vi "Automatic.vi"() -> ()   [LabVIEW 2015]
uses:
  <vilib>/myRIO/Instrument Drivers/Onboard IO/PWM/typedefs/PWM Reference.ctl
  <vilib>/myRIO/Common/Instrument Driver Framework/Utilities/typedefs/myRIO Generic Hardware Reference.ctl
  <vilib>/myRIO/Common/Instrument Driver Framework/Utilities/typedefs/Hardware Version Enum.ctl
  <vilib>/myRIO/Common/Instrument Driver Framework/Utilities/typedefs/myRIO v1.0 Reference.ctl
  <vilib>/myRIO/Common/Instrument Driver Framework/Utilities/typedefs/Generic FPGA Reference.ctl
  <vilib>/myRIO/Common/Instrument Driver Framework/myRIO v1.0/PWM/typedefs/PWM Channels Enum.ctl
  <vilib>/myRIO/Instrument Drivers/Onboard IO/PWM/typedefs/PWM Configuration.ctl
  <vilib>/userdefined/High Color/nirio_resource_hc.ctl
  <vilib>/myRIO/Instrument Drivers/Onboard IO/DIO/typedefs/DIO Reference.ctl
  <vilib>/myRIO/Common/Instrument Driver Framework/myRIO v1.0/DIO/typedefs/DIO Channels List.ctl
  <vilib>/myRIO/Common/Instrument Driver Framework/myRIO v1.0/DIO/typedefs/DIO Channels Enum.ctl
  <vilib>/myRIO/Common/Instrument Driver Framework/Utilities/vis/Is FPGA Ref Available.vi
  <vilib>/myRIO/Common/Instrument Driver Framework/myRIO v1.0/DIO/vis/myRIO v1.1 Open DIO.vi
  <vilib>/myRIO/Instrument Drivers/Onboard IO/DIO/vis/Write.vi
  <vilib>/myRIO/Common/Instrument Driver Framework/myRIO v1.0/PWM/vis/myRIO v1.1 Open PWM.vi
  <vilib>/myRIO/Common/Instrument Driver Framework/Utilities/vis/Validate Channels.vi
  <vilib>/myRIO/Common/Instrument Driver Framework/myRIO v1.0/DIO/vis/myRIO v1.0 Reserve DIO.vi
  <vilib>/myRIO/Common/Instrument Driver Framework/myRIO v1.0/PWM/vis/myRIO v1.0 Reserve PWM.vi
  <vilib>/myRIO/Instrument Drivers/Onboard IO/PWM/vis/Set Duty Cycle and Frequency.vi
  <vilib>/myRIO/Common/Instrument Driver Framework/myRIO v1.0/PWM/vis/myRIO v1.0 Close PWM.vi
  <vilib>/myRIO/Common/Instrument Driver Framework/myRIO v1.0/UART/vis/myRIO v1.0 Close UART.vi
  <vilib>/myRIO/Common/Instrument Driver Framework/myRIO v1.0/Resource Manager/vis/myRIO v1.0 Reserve Channel List.vi
  <vilib>/myRIO/Common/Instrument Driver Framework/myRIO v1.0/DIO/vis/myRIO v1.0 Build MUX Configuration DIO.vi
  <vilib>/myRIO/Common/Instrument Driver Framework/myRIO v1.0/PWM/vis/myRIO v1.0 Build MUX Configuration PWM.vi
  <vilib>/myRIO/Common/Instrument Driver Framework/myRIO v1.0/PWM/vis/myRIO v1.0 Unreserve PWM.vi
  <vilib>/myRIO/Common/Instrument Driver Framework/myRIO v1.0/Resource Manager/vis/myRIO v1.0 Reserve Channel.vi
  <vilib>/myRIO/Common/Instrument Driver Framework/myRIO v1.0/Resource Manager/vis/myRIO v1.0 Unreserve Channel.vi
  <vilib>/myRIO/Common/Instrument Driver Framework/myRIO v1.0/Resource Manager/vis/myRIO v1.0 Create Configuration List.vi
  <vilib>/myRIO/Common/Instrument Driver Framework/myRIO v1.0/Resource Manager/vis/myRIO v1.0 Unreserve Channel List.vi
  <vilib>/myRIO/Common/Instrument Driver Framework/myRIO v1.0/Resource Manager/vis/myRIO v1.0 Build Mutex Name.vi
  <vilib>/Utility/VariantDataType/GetNumericInfo.vi
  <vilib>/Utility/error.llb/Error Cluster From Error Code.vi
  <vilib>/myRIO/Common/Instrument Driver Framework/myRIO v1.0/myRIO v1.1 Open.vi
  <vilib>/myRIO/Common/Instrument Driver Framework/Utilities/vis/IO Manager.vi
  <vilib>/myRIO/Common/Instrument Driver Framework/Utilities/vis/Configuration Manager.vi
  <vilib>/myRIO/Common/Instrument Driver Framework/myRIO v1.0/Resource Manager/vis/myRIO v1.0 Configure IO.vi
  <vilib>/myRIO/Common/Instrument Driver Framework/myRIO v1.0/myRIO v1.0 Close.vi
  <vilib>/myRIO/Common/Instrument Driver Framework/myRIO v1.0/PWM/vis/myRIO v1.0 Write PWM.vi
  <vilib>/myRIO/Common/Instrument Driver Framework/myRIO v1.0/PWM/vis/myRIO v1.0 Shutdown PWM.vi
  <vilib>/myRIO/Common/Instrument Driver Framework/Utilities/vis/FPGA Ref Manager.vi
  <vilib>/myRIO/Common/Instrument Driver Framework/myRIO v1.0/myRIO v1.0 Reset FPGA.vi
  <vilib>/myRIO/Common/Instrument Driver Framework/myRIO v1.0/IRQ/vis/myRIO v1.0 IRQ Info FGV.vi
  <vilib>/myRIO/Common/Instrument Driver Framework/myRIO v1.0/IRQ/vis/myRIO v1.0 Timer IRQ Info FGV.vi
  <vilib>/myRIO/Common/Instrument Driver Framework/myRIO v1.0/IRQ/vis/myRIO v1.0 ISR Agent.vi
  <vilib>/myRIO/Common/Instrument Driver Framework/myRIO v1.0/DIO/vis/myRIO v1.0 Write DIO.vi
  <vilib>/myRIO/Instrument Drivers/Onboard IO/PWM/vis/myRIO PWM Open.xnode
  <vilib>/myRIO/Express VI/Onboard Devices/LED/LED Express VI.xnode
  <vilib>/myRIO/Instrument Drivers/Onboard IO/DIO/vis/myRIO DIO Open.xnode
  <vilib>/myRIO/Instrument Drivers/Onboard IO/PWM/PWM.lvlib
  <vilib>/myRIO/Instrument Drivers/Utilities/Utilities.lvlib
  <vilib>/myRIO/Instrument Drivers/Onboard IO/DIO/DIO.lvlib
panel:
  in  "Automate":bool
  in  "Water Spill Guard":bool
  out "Sensor Pin":T1
  out "Gripper Pin":T1
  out "Pour Pin":T1
  in  "Pour":bool
  out "Information":string="Pour"
  out "Counter":dbl=1.0
  out "New Duty Cycle":dbl=nan
  in  "Stop [ESC]":bool
  in  "Gripper":bool
  out "Water Detected":bool
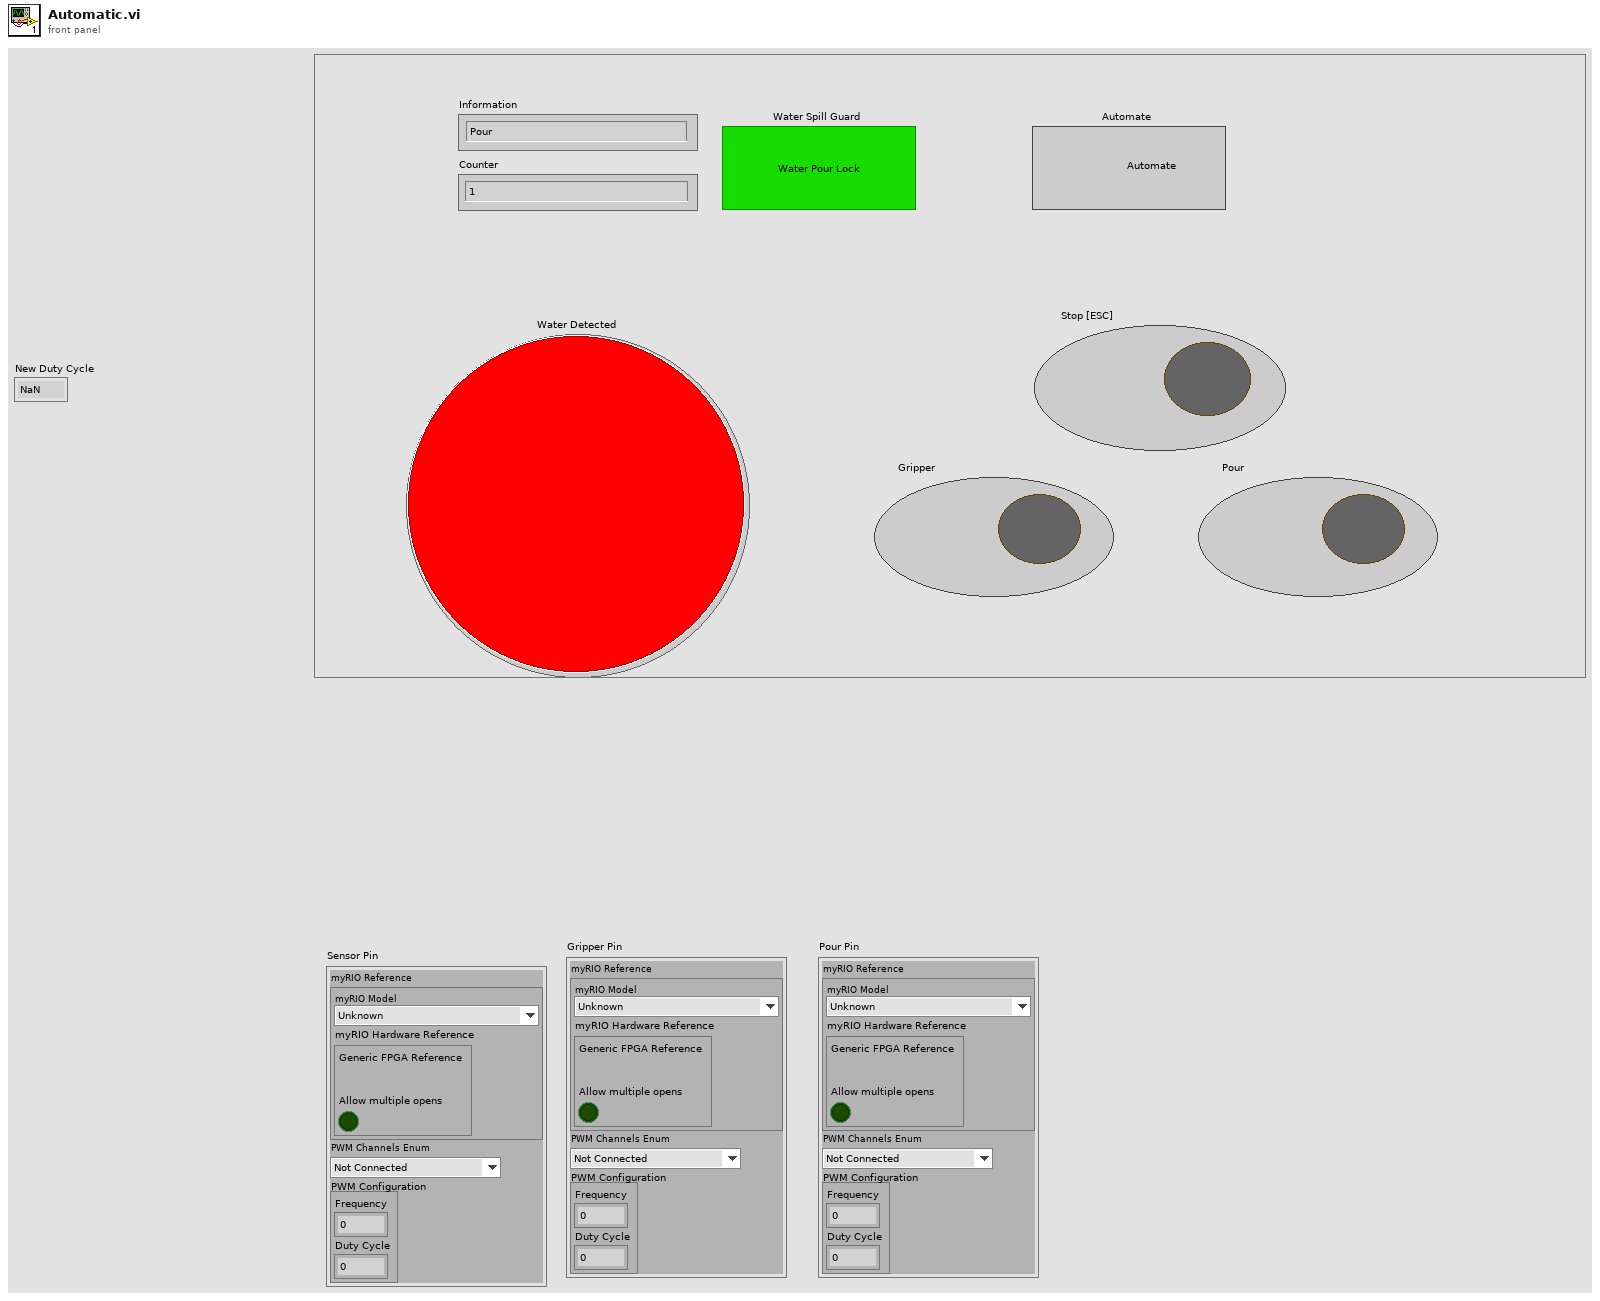
[diagram p1: front panel]
types:
  T1 = typedef "PWM.lvlib/PWM Reference.ctl" = cluster{"myRIO Reference":T2, "PWM Channels Enum":T6, "PWM Configuration":T7}
  T2 = typedef "myRIO Generic Hardware Reference.ctl" = cluster{"myRIO Model":T3, "myRIO Hardware Reference":T4}
  T3 = typedef "Hardware Version Enum.ctl" = enum16{"Unknown", "myRIO-1900", "myRIO-1950", "roboRIO"}
  T4 = typedef "myRIO v1.0 Reference.ctl" = cluster{"Generic FPGA Reference":T5, "Allow multiple opens":bool}
  T5 = typedef "Generic FPGA Reference.ctl" = refnum<k20>
  T6 = typedef "PWM Channels Enum.ctl" = enum16{"Not Connected", "C/PWM0", "C/PWM1", "A/PWM0", "A/PWM1", "A/PWM2", "B/PWM0", "B/PWM1", "B/PWM2", "PWM/PWM0", "PWM/PWM1", "PWM/PWM2", "PWM/PWM3", "PWM/PWM4", "PWM/PWM5", "PWM/PWM6", "PWM/PWM7", "PWM/PWM8", "PWM/PWM9"}
  T7 = typedef "PWM.lvlib/PWM Configuration.ctl" = cluster{"Frequency":dbl, "Duty Cycle":dbl}
  T8 = typedef "nirio_resource_hc.ctl" = tag
  T9 = typedef "DIO.lvlib/DIO Reference.ctl" = cluster{"myRIO Reference":T2, "DIO Channels List":T10}
  T10 = typedef "DIO Channels List.ctl" = T11[]
  T11 = typedef "DIO Channels Enum.ctl" = enum16{"Not Connected", "C/DIO0", "C/DIO1", "C/DIO2", "C/DIO3", "C/DIO4", "C/DIO5", "C/DIO6", "C/DIO7", "A/DIO0", "A/DIO1", "A/DIO2", "A/DIO3", "A/DIO4", "A/DIO5", "A/DIO6", "A/DIO7", "A/DIO8", "A/DIO9", "A/DIO10", "A/DIO11", "A/DIO12", "A/DIO13", "A/DIO14", "A/DIO15", "B/DIO0", "B/DIO1", "B/DIO2", "B/DIO3", "B/DIO4", "B/DIO5", "B/DIO6", "B/DIO7", "B/DIO8", "B/DIO9", "B/DIO10", "B/DIO11", "B/DIO12", "B/DIO13", "B/DIO14", "B/DIO15", "LED0", "LED1", "LED2", "LED3", "Button0", "DIO/DIO0", "DIO/DIO1", "DIO/DIO2", "DIO/DIO3", "DIO/DIO4", "DIO/DIO5", "DIO/DIO6", "DIO/DIO7", "DIO/DIO8", "DIO/DIO9", "SPI/CS0", "SPI/CS1", "SPI/CS2", "SPI/CS3", "LED RADIO (Green)", "LED RADIO (Red)", "LED COMM (Green)", "LED COMM (Red)", "LED MODE (Green)", "LED MODE (Red)"}
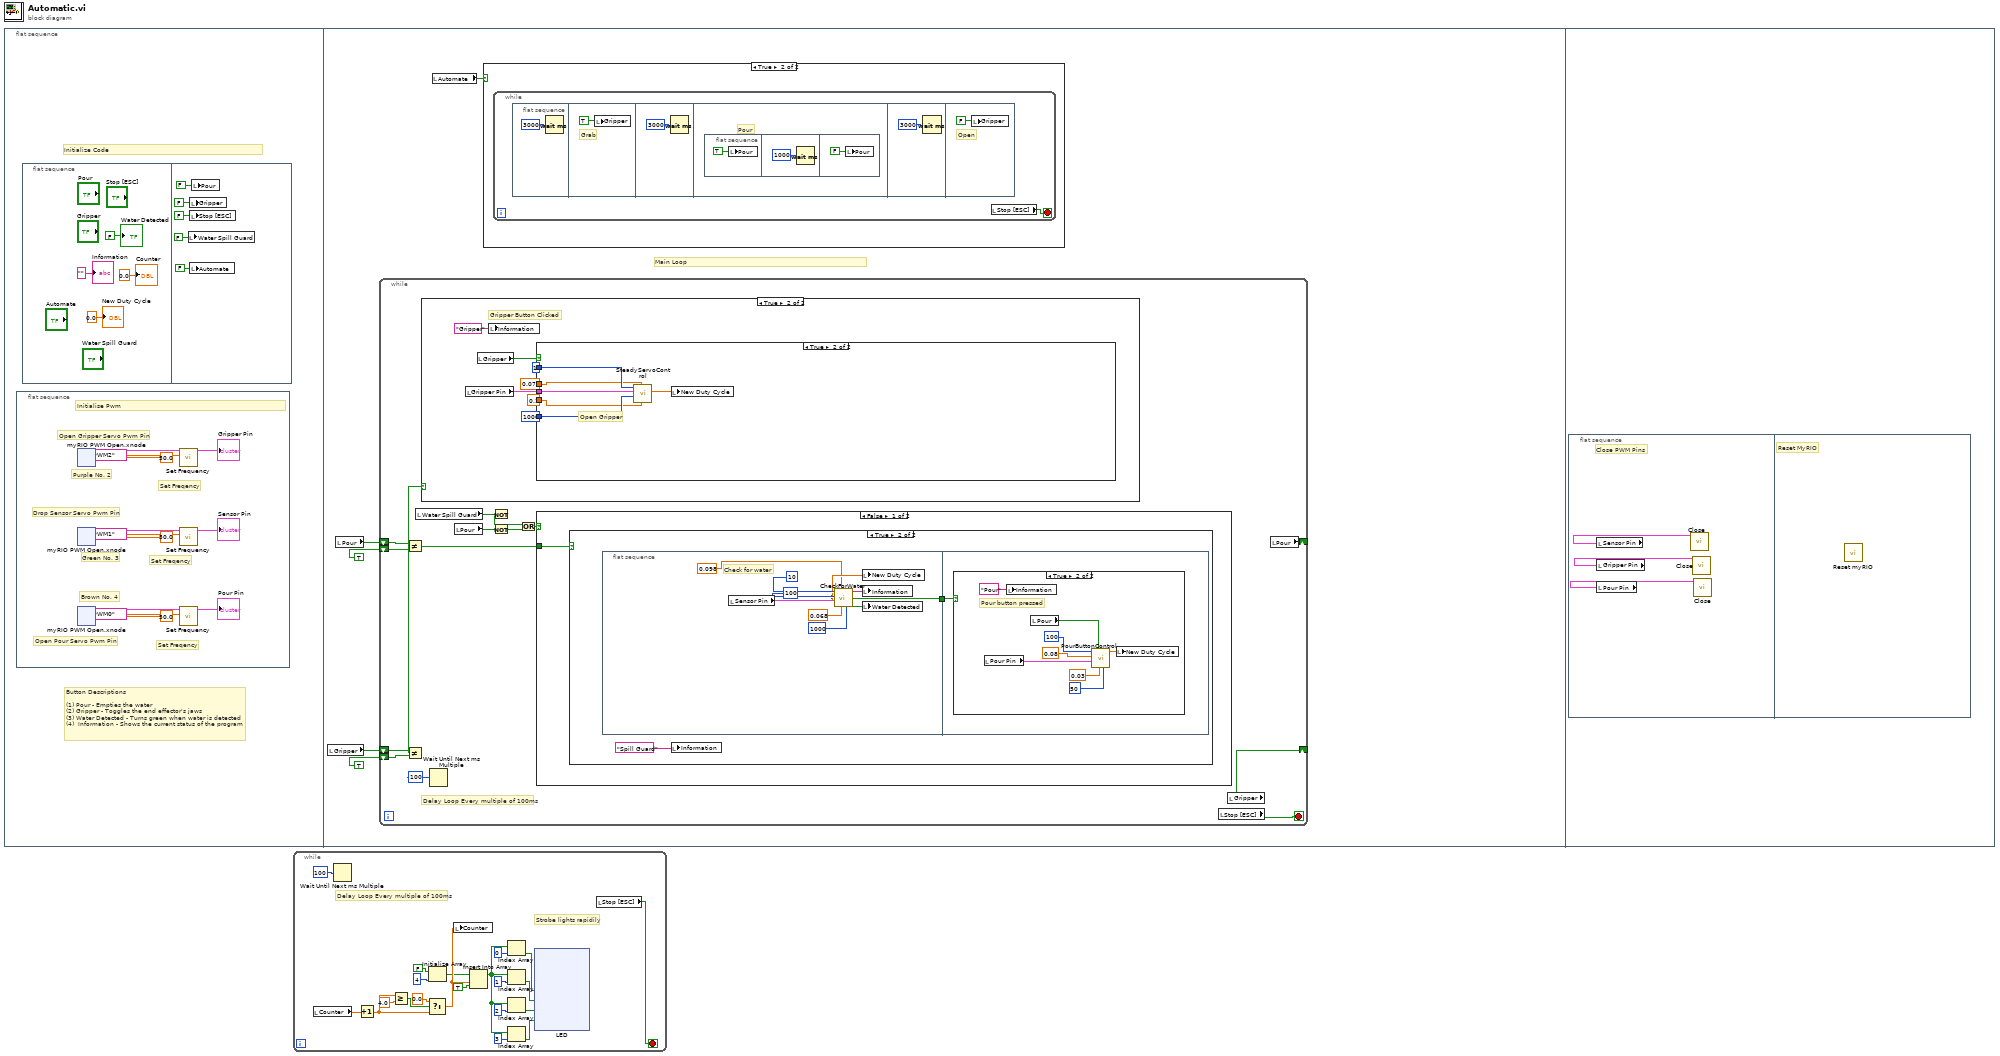
[diagram p0: block diagram]
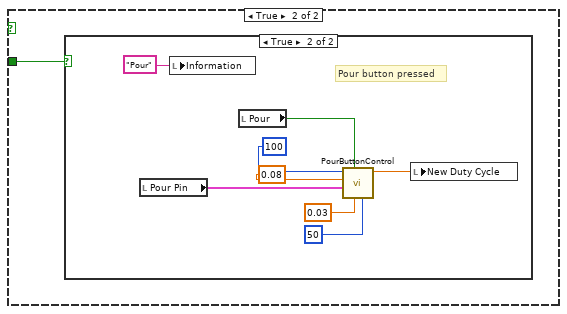
[diagram p5: hidden frame]
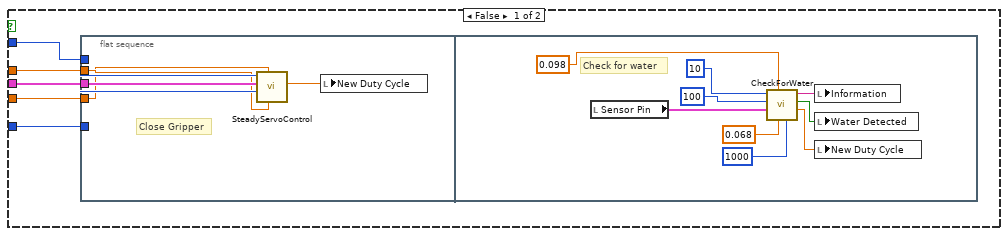
[diagram p8: hidden frame]
diagram:
  n1 = flat-sequence {
    frame #0 {
      # "Button Descriptions\n\n(1) Pour - Empties the water\n(2) Gripper - Toggles the end effector's jaws\n(3) Water Detected - Turns green when water is detected\n(4)  Information - Shows the current status of the program"
      # "Initialize Code"
      n2 = flat-sequence {
        frame #0 {
          # "Green No. 3"
          # "Set Freqency"
          # "Drop Sensor Servo Pwm Pin"
          # "Initialise Pwm"
          # "Purple No. 2"
          # "Set Freqency"
          # "Open Gripper Servo Pwm Pin"
          # "Set Freqency"
          # "Brown No. 4"
          # "Open Pour Servo Pwm Pin"
          n3 = xnode "myRIO PWM Open.xnode"("Channel Name"=tag "A/PWM2") -> ("PWM Ref Out"=w7:T1)  [unwired: 2 in, 1 out]
          n4 = xnode "myRIO PWM Open.xnode"("Channel Name"=tag "A/PWM1") -> ("PWM Ref Out"=w2:T1)  [unwired: 2 in, 1 out]
          n5 = xnode "myRIO PWM Open.xnode"("Channel Name"=tag "A/PWM0") -> ("PWM Ref Out"=w10:T1)  [unwired: 2 in, 1 out]
          n6 = call <vilib>:"Set Frequency.vi"("Frequency [Hz]"=50.0, "PWM Ref In"=w7) -> ("PWM Ref Out"=→"Gripper Pin":T1)  [unwired: 7 in, 1 out]
          n7 = call <vilib>:"Set Frequency.vi"("Frequency [Hz]"=50.0, "PWM Ref In"=w2) -> ("PWM Ref Out"=→"Sensor Pin":T1)  [unwired: 7 in, 1 out]
          n8 = call <vilib>:"Set Frequency.vi"("Frequency [Hz]"=50.0, "PWM Ref In"=w10) -> ("PWM Ref Out"=→"Pour Pin":T1)  [unwired: 7 in, 1 out]
        }
      }
      n9 = flat-sequence {
        frame #0 {
          "Water Detected" <- FALSE ("Water Detected")
          "Counter" <- 0.0 ("Counter")
          "Information" <- "" ("Information")
          "New Duty Cycle" <- 0.0 ("New Duty Cycle")
        }
        frame #1 {
          n10 = local write "Water Spill Guard"(FALSE ("Water Spill Guard")) -> ()
          n11 = local write "Gripper"(FALSE ("Pour")) -> ()
          n12 = local write "Stop [ESC]"(FALSE ("Pour")) -> ()
          n13 = local write "Automate"(FALSE ("Automate")) -> ()
          n14 = local write "Pour"(FALSE ("Pour")) -> ()
        }
      }
    }
    frame #1 {
      # "Main Loop"
      n15 = local read "Gripper"() -> (w74:bool)
      n16 = local read "Pour"() -> (w72:bool)
      n17 = while {
        shift-right: [w98] -> _
        shift-left: w74 -> [w96]
        shift-left: TRUE ("Gripper") -> [w95]
        shift-right: [w90] -> _
        shift-left: w72 -> [w92]
        shift-left: TRUE ("Pour") -> [w91]
        stop <- w94 stop-if-true
        # "Delay Loop Every multiple of 100ms"
        n18 = Not Equal?(x=w92, y=w91) -> (x != y?=w84:bool)
        n19 = Not Equal?(x=w96, y=w95) -> (x != y?=w97:bool)
        n20 = local read "Water Spill Guard"() -> (w86:bool)
        n21 = case shown="True" w97 {
          frame False {
          }
          frame True {
            # "Gripper Button Clicked"
            n22 = local read "Gripper Pin"() -> (w133:T1)
            n23 = local read "Gripper"() -> (w134:bool)
            n24 = local write "Information"("Gripper" ("Information")) -> ()
            n25 = case shown="True" w134 {
              tunnel: w133 -> [w140 w158]
              tunnel: u32 1 ("Wait Time") -> [w139 w160]
              tunnel: 1000 ("Steps") -> [w138 w159]
              tunnel: 0.074 ("Prev Duty Cycle") -> [w137 w157]
              tunnel: 0.1 ("New Duty Cycle") -> [w136 w156]
              frame False {
                n26 = flat-sequence {
                  tunnel: w140 -> [w145]
                  tunnel: w139 -> [w144]
                  tunnel: w138 -> [w143]
                  tunnel: w137 -> [w142]
                  tunnel: w136 -> [w141]
                  frame #0 {
                    # "Close Gripper"
                    n27 = call "SteadyServoControl.vi"("New Duty Cycle"=w142, "Prev Duty Cycle"=w141, "Steps"=w143, "PWM Ref Out in"=w145, "Wait Time"=w144) -> ("Numeric"=w146:dbl)  [unwired: 5 in, 1 out]
                    n28 = local write "New Duty Cycle"(w146) -> ()
                  }
                  frame #1 {
                    # "Check for water"
                    n29 = local read "Sensor Pin"() -> (w148:T1)
                    n30 = call "CheckForWater.vi"("milliseconds to wait"=u32 1000, "f"=0.068, "t"=0.098, "Sensor Pin"=w148, "Steps"=100, "Wait Time"=u32 10) -> ("Numeric"=w147:dbl, "A/DIO0 (Pin 11)"=w153:bool, "Information"=w155:string)  [unwired: 3 in]
                    n31 = local write "Information"(w155) -> ()
                    n32 = local write "Water Detected"(w153) -> ()
                    n33 = local write "New Duty Cycle"(w147) -> ()
                  }
                }
              }
              frame True {
                # "Open Gripper"
                n34 = call "SteadyServoControl.vi"("New Duty Cycle"=w156, "Prev Duty Cycle"=w157, "Steps"=w159, "PWM Ref Out in"=w158, "Wait Time"=w160) -> ("Numeric"=w161:dbl)  [unwired: 5 in, 1 out]
                n35 = local write "New Duty Cycle"(w161) -> ()
              }
            }
          }
        }
        n36 = Wait Until Next ms Multiple(millisecond multiple=u32 100) -> ()  [unwired: 1 out]
        n37 = local read "Pour"() -> (w89:bool)
        n38 = Not(x=w86) -> (.not. x?=w85:bool)
        n39 = Not(x=w89) -> (.not. x?=w88:bool)
        n40 = Or(x=w85, y=w88) -> (x .or. y?=w87:bool)
        n41 = case shown="False" w87 {
          tunnel: w84 -> [w99 w120]
          frame False {
            n42 = case shown="True" w99 {
              frame False {
              }
              frame True {
                n43 = flat-sequence {
                  tunnel: [w102] -> w100
                  tunnel: w100 -> [w111]
                  frame #0 {
                    # "Check for water"
                    n44 = local read "Sensor Pin"() -> (w105:T1)
                    n45 = call "CheckForWater.vi"("milliseconds to wait"=u32 1000, "f"=0.068, "t"=0.098, "Sensor Pin"=w105, "Steps"=100, "Wait Time"=u32 10) -> ("Numeric"=w104:dbl, "A/DIO0 (Pin 11)"=w102:bool, "Information"=w110:string)  [unwired: 3 in]
                    n46 = local write "New Duty Cycle"(w104) -> ()
                    n47 = local write "Information"(w110) -> ()
                    n48 = local write "Water Detected"(w102) -> ()
                  }
                  frame #1 {
                    n49 = case shown="True" w111 {
                      frame False {
                      }
                      frame True {
                        # "Pour button pressed"
                        n50 = local read "Pour Pin"() -> (w114:T1)
                        n51 = local write "Information"("Pour" ("Information")) -> ()
                        n52 = local read "Pour"() -> (w113:bool)
                        n53 = call "PourButtonControl.vi"("Steps"=50, "Prev Duty Cycle"=0.03, "Pour"=w113, "Pour Pin"=w114, "New Duty Cycle"=0.08, "Wait Time"=u32 100) -> ("Numeric"=w119:dbl)  [unwired: 5 in]
                        n54 = local write "New Duty Cycle"(w119) -> ()
                      }
                    }
                  }
                }
                n55 = local write "Information"("Spill Guard" ("Information")) -> ()
              }
            }
          }
          frame True {
            n56 = case shown="True" w120 {
              frame False {
              }
              frame True {
                # "Pour button pressed"
                n57 = local read "Pour Pin"() -> (w126:T1)
                n58 = local write "Information"("Pour" ("Information")) -> ()
                n59 = local read "Pour"() -> (w127:bool)
                n60 = call "PourButtonControl.vi"("Steps"=50, "Prev Duty Cycle"=0.03, "Pour"=w127, "Pour Pin"=w126, "New Duty Cycle"=0.08, "Wait Time"=u32 100) -> ("Numeric"=w121:dbl)  [unwired: 5 in]
                n61 = local write "New Duty Cycle"(w121) -> ()
              }
            }
          }
        }
        n62 = local read "Stop [ESC]"() -> (w94:bool)
        n63 = local read "Gripper"() -> (w98:bool)
        n64 = local read "Pour"() -> (w90:bool)
      }
      n65 = local read "Automate"() -> (w70:bool)
      n66 = case shown="True" w70 {
        frame False {
        }
        frame True {
          n67 = while {
            stop <- w75 stop-if-true
            n68 = flat-sequence {
              frame #0 {
                n69 = Wait (ms)(milliseconds to wait=u32 3000) -> ()  [unwired: 1 out]
              }
              frame #1 {
                # "Grab"
                n70 = local write "Gripper"(TRUE ("Gripper")) -> ()
              }
              frame #2 {
                n71 = Wait (ms)(milliseconds to wait=u32 3000) -> ()  [unwired: 1 out]
              }
              frame #3 {
                # "Pour"
                n72 = flat-sequence {
                  frame #0 {
                    n73 = local write "Pour"(TRUE ("Pour")) -> ()
                  }
                  frame #1 {
                    n74 = Wait (ms)(milliseconds to wait=u32 1000) -> ()  [unwired: 1 out]
                  }
                  frame #2 {
                    n75 = local write "Pour"(FALSE ("Pour")) -> ()
                  }
                }
              }
              frame #4 {
                n76 = Wait (ms)(milliseconds to wait=u32 3000) -> ()  [unwired: 1 out]
              }
              frame #5 {
                # "Open"
                n77 = local write "Gripper"(FALSE ("Gripper")) -> ()
              }
            }
            n78 = local read "Stop [ESC]"() -> (w75:bool)
          }
        }
      }
    }
    frame #2 {
      n79 = flat-sequence {
        frame #0 {
          # "Close PWM Pins"
          n80 = local read "Sensor Pin"() -> (w162:T1)
          n81 = local read "Gripper Pin"() -> (w163:T1)
          n82 = local read "Pour Pin"() -> (w164:T1)
          n83 = call <vilib>:"Close.vi"("PWM Ref In"=w162) -> ()  [unwired: 10 in, 1 out]
          n84 = call <vilib>:"Close.vi"("PWM Ref In"=w163) -> ()  [unwired: 10 in, 1 out]
          n85 = call <vilib>:"Close.vi"("PWM Ref In"=w164) -> ()  [unwired: 10 in, 1 out]
        }
        frame #1 {
          # "Reset MyRIO"
          n86 = call <vilib>:"Reset myRIO.vi"() -> ()  [unwired: 11 in, 1 out]
        }
      }
    }
  }
  n87 = while {
    stop <- w166 stop-if-true
    # "Delay Loop Every multiple of 100ms"
    # "Strobe lights rapidily"
    n88 = local read "Counter"() -> (w185:dbl)
    n89 = Wait Until Next ms Multiple(millisecond multiple=u32 100) -> ()  [unwired: 1 out]
    n90 = Increment(x=w185) -> (x+1=w170:dbl)
    n91 = Greater Or Equal?(x=w170, y=4.0) -> (x >= y?=w168:bool)
    n92 = Select(t=0.0, s=w168, f=w170) -> (s? t:f=w184:dbl)
    n93 = Initialize Array(FALSE, 4 ("dimension size")) -> (w181:bool[])
    n94 = local write "Counter"(w184) -> ()
    n95 = Insert Into Array(array=w181, index=w184, new element=TRUE ("new element/subarray")) -> (w182:bool[])
    n96 = Index Array(array=w182, index=0) -> (element=w172:bool)
    n97 = Index Array(array=w182, index=1) -> (element=w178:bool)
    n98 = Index Array(array=w182, index=2) -> (element=w179:bool)
    n99 = Index Array(array=w182, index=3) -> (element=w180:bool)
    n100 = xnode "LED"("LED0"=w172, "LED1"=w178, "LED2"=w179, "LED3"=w180) -> ()  [unwired: 1 in, 1 out]
    n101 = local read "Stop [ESC]"() -> (w166:bool)
  }
